vi "Destroy.vi"(8 "error in (no error)":errorcluster, 11 "Event Registration Refnum":refnum<event-registration>) -> (0 "error out":errorcluster)   [LabVIEW 2017, in "WebServiceImporter.lvlib" / "Main Panel.lvlib" / "Events.lvlib"]
uses:
  <vilib>/Platform/WebService/Main Panel/Events/Events.lvlib
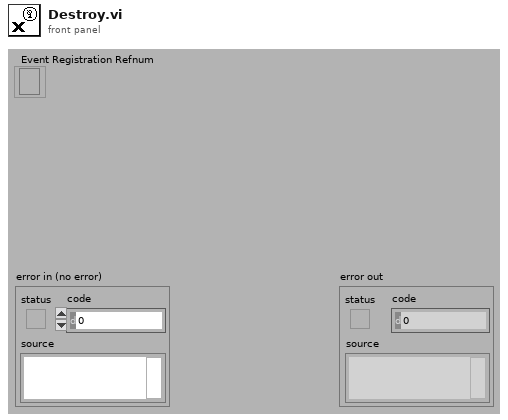
[diagram p1: front panel]
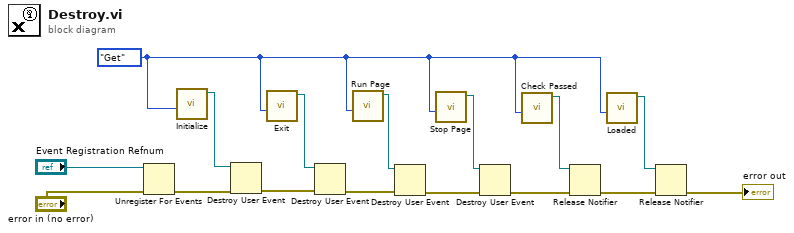
[diagram p0: block diagram]
diagram:
  w2 = enum16{"Get", "Set"}."Get" ("Operation")
  n1 = Unregister For Events(event registration refnum="Event Registration Refnum", error in="error in (no error)") -> (error out=w15:errorcluster)
  n2 = call <vilib>:"Initialize.vi"("Operation"=w2) -> ("user event out"=w14:refnum<user-event>)  [unwired: 10 in]
  n3 = Destroy User Event(user event=w14, error in=w15) -> (error out=w13:errorcluster)
  n4 = call <vilib>:"Exit.vi"("Operation"=w2) -> ("user event (out)"=w12:refnum<user-event>)  [unwired: 10 in]
  n5 = Destroy User Event(user event=w12, error in=w13) -> (error out=w11:errorcluster)
  n6 = call <vilib>:"Run Page.vi"("Operation"=w2) -> ("user event  (out)"=w10:refnum<user-event>)  [unwired: 10 in]
  n7 = Destroy User Event(user event=w10, error in=w11) -> (error out=w9:errorcluster)
  n8 = call <vilib>:"Stop Page.vi"("Operation"=w2) -> ("user event (out)"=w8:refnum<user-event>)  [unwired: 10 in]
  n9 = Destroy User Event(user event=w8, error in=w9) -> (error out=w7:errorcluster)
  n10 = call <vilib>:"Check Passed.vi"("Operation"=w2) -> ("notifier  (out)"=w4:refnum<notifier>)  [unwired: 9 in, 1 out]
  n11 = Release Notifier(notifier=w4, error in (no error)=w7) -> (error out=w6:errorcluster)  [unwired: 1 in, 2 out]
  n12 = call <vilib>:"Loaded.vi"("Operation"=w2) -> ("notifier (out)"=w3:refnum<notifier>)  [unwired: 10 in]
  n13 = Release Notifier(notifier=w3, error in (no error)=w6) -> (error out=→"error out":errorcluster)  [unwired: 1 in, 2 out]
